vi "GenerateFilenames_2P.vi"(7 "path":path) -> (0 "WebCam Path":path, 1 "Basler Path":path, 2 "TDMS Path":path, 3 "MScan Path":path, 5 "Analog file name":string="F:\\Data\\130725_14_35_2625")   [LabVIEW 2020]
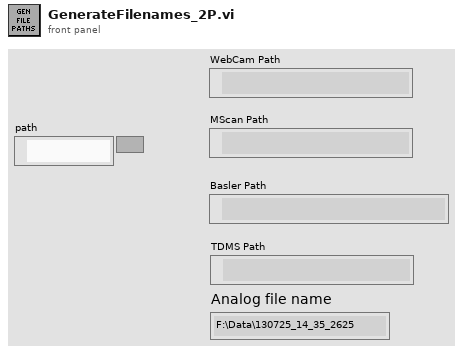
[diagram p1: front panel]
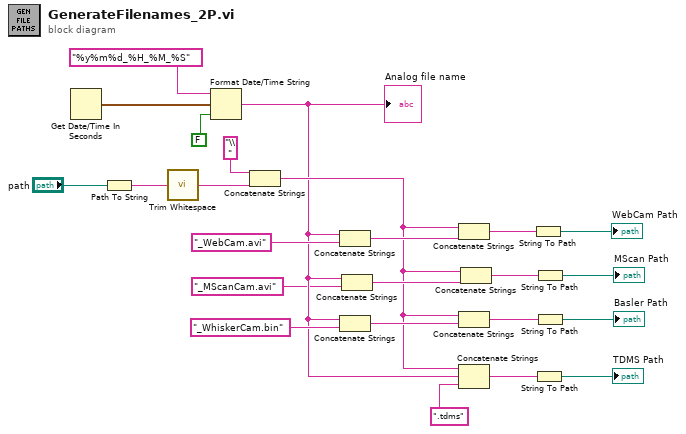
[diagram p0: block diagram]
diagram:
  n1 = Get Date/Time In Seconds() -> (seconds since 1Jan1904=w23:timestamp)
  n2 = Path To String(path="path") -> (string=w11:string)
  n3 = call <vilib>:"Trim Whitespace.vi"("string"=w11) -> ("trimmed string"=w9:string)  [unwired: 1 in]
  n4 = Format Date/Time String(time format string (%c)="%y%m%d_%H_%M_%S", seconds (now)=w23, UTC format=FALSE) -> (date/time string=w2:string)
  "Analog file name" <- w2
  n5 = Concatenate Strings(w9, "\\" ("string")) -> (w3:string)
  n6 = Concatenate Strings(w2, "_WebCam.avi") -> (w21:string)
  n7 = Concatenate Strings(w2, "_WhiskerCam.bin" ("string")) -> (w18:string)
  n8 = Concatenate Strings(w2, "_MScanCam.avi") -> (w6:string)
  n9 = Concatenate Strings(w3, w21) -> (w20:string)
  n10 = Concatenate Strings(w3, w18) -> (w17:string)
  n11 = Concatenate Strings(w3, w2, ".tdms" ("string")) -> (w12:string)
  n12 = Concatenate Strings(w3, w6) -> (w5:string)
  n13 = String To Path(string=w20) -> (path=→"WebCam Path":path)
  n14 = String To Path(string=w12) -> (path=→"TDMS Path":path)
  n15 = String To Path(string=w5) -> (path=→"MScan Path":path)
  n16 = String To Path(string=w17) -> (path=→"Basler Path":path)
